vi "Read UI Constants.vi"(8 "error in":errorcluster, 11 "CFG File Refnum in":T2) -> (0 "error out":errorcluster, 2 "MHL Configuration":T1, 3 "CFG File Refnum out":T2)   [LabVIEW 2014]
uses:
  <vilib>/Utility/config.llb/Config Data RefNum.ctl
  controls/MHL Configuration.ctl
  Boiler System Globals.vi
  <vilib>/Utility/config.llb/Read Key (Double).vi
  <vilib>/Utility/error.llb/Error Cluster From Error Code.vi
  <vilib>/ErrorRing/Error Ring.xnode
  <vilib>/Utility/config.llb/NI_LVConfig.lvlib
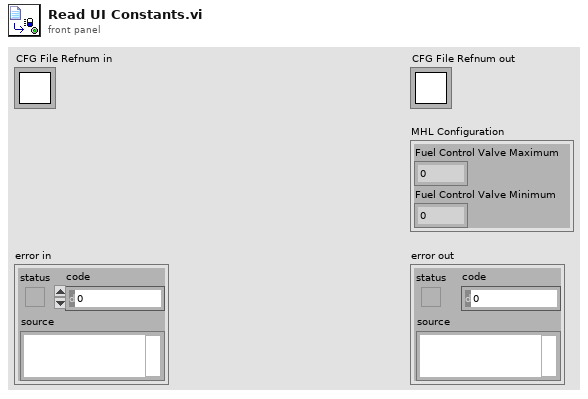
[diagram p1: front panel]
types:
  T1 = typedef "MHL Configuration.ctl" = cluster{"Fuel Control Valve Maximum":dbl, "Fuel Control Valve Minimum":dbl}
  T2 = typedef "NI_LVConfig.lvlib/Config Data RefNum.ctl" = refnum<k1>
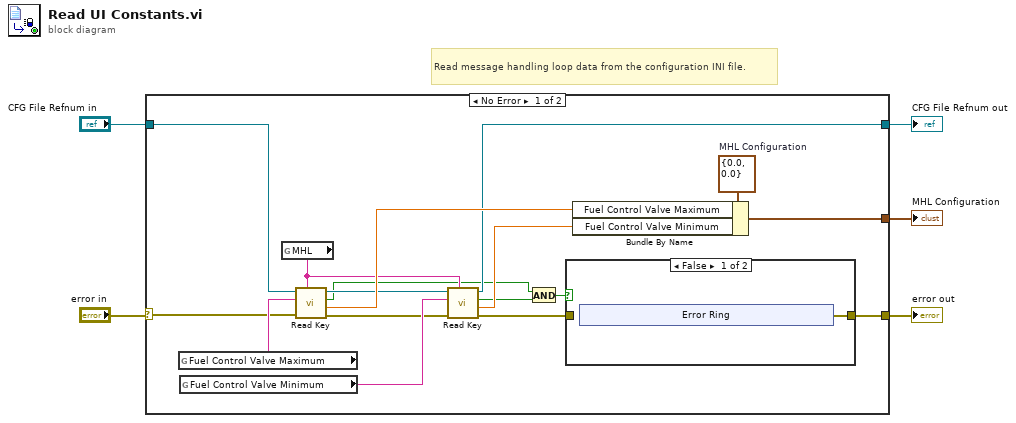
[diagram p0: block diagram]
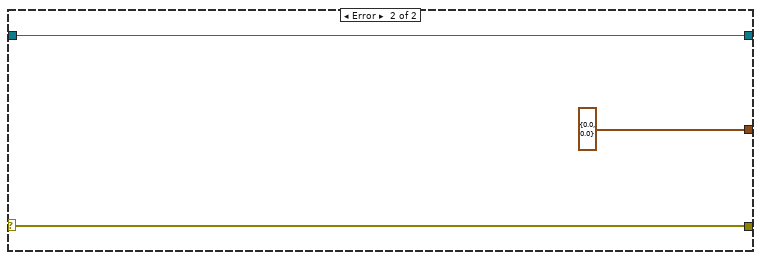
[diagram p3: hidden frame]
diagram:
  # "Read message handling loop data from the configuration INI file."
  n1 = case shown="No Error" "error in" {
    selector: "error in" -> [w20 w31]
    tunnel: "CFG File Refnum in" -> [w21 w32]
    tunnel: [w7 w31] -> w4
    tunnel: [w12 w32] -> w3
    tunnel: [w17 T1 {"Fuel Control Valve Maximum"=0.0, "Fuel Control Valve Minimum"=0.0} ("MHL Configuration Data")] -> w1
    frame No Error {
      w19 = T1 {"Fuel Control Valve Maximum"=0.0, "Fuel Control Valve Minimum"=0.0}  # MHL Configuration
      n2 = global read "Boiler System Globals.vi" "Fuel Control Valve Maximum"() -> (w22:string)
      n3 = global read "Boiler System Globals.vi" "Fuel Control Valve Minimum"() -> (w16:string)
      n4 = global read "Boiler System Globals.vi" "MHL"() -> (w14:string)
      n5 = call-poly <vilib>:"Read Key.vi"("section"=w14, "error in (no error)"=w20, "key"=w22, "refnum"=w21) -> ("error out"=w15:errorcluster, "value"=w18:dbl, "found?"=w8:bool, "refnum out"=w13:T2)  [unwired: 4 in]
      n6 = call-poly <vilib>:"Read Key.vi"("section"=w14, "error in (no error)"=w15, "key"=w16, "refnum"=w13) -> ("error out"=w6:errorcluster, "value"=w11:dbl, "found?"=w9:bool, "refnum out"=w12:T2)  [unwired: 4 in]
      n7 = And(x=w8, y=w9) -> (x .and. y?=w10:bool)
      n8 = case shown="False" w10 {
        tunnel: [w23 w29] -> w7
        tunnel: w6 -> [_ w29]
        frame False {
          n9 = xnode "Error Ring"() -> ("error out"=w23:errorcluster)
        }
        frame True {
        }
      }
      n10 = Bundle By Name(cluster=w19, "Fuel Control Valve Maximum"=w18, "Fuel Control Valve Minimum"=w11) -> (w17:T1)
    }
    frame Error {
    }
  }
  "error out" <- w4
  "CFG File Refnum out" <- w3
  "MHL Configuration" <- w1
